vi "convert--chessboard_index to chess_square (chess notation).vi"(1 "chessboard_index":T4) -> (0 "chess_square (chess notation)":T1)   [LabVIEW 2020, in "core.lvlib"]
uses:
  core.lvlib
  core_data/chessboard_index.ctl
  core_data/chess_square--chess notation.ctl
  core_data/file--enum.ctl
  core_data/rank--enum.ctl
  core_data/core_data.lvlib
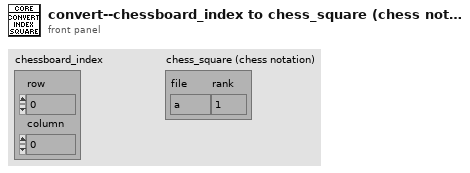
[diagram p1: front panel]
types:
  T1 = typedef "core.lvlib/core_data.lvlib/chess_square--chess notation.ctl" = cluster{"file":T2, "rank":T3}
  T2 = typedef "core.lvlib/core_data.lvlib/file--enum.ctl" = enum16{"a", "b", "c", "d", "e", "f", "g", "h"}
  T3 = typedef "core.lvlib/core_data.lvlib/rank--enum.ctl" = enum16{"1", "2", "3", "4", "5", "6", "7", "8"}
  T4 = typedef "core.lvlib/core_data.lvlib/chessboard_index.ctl" = cluster{"row":u8, "column":u8}
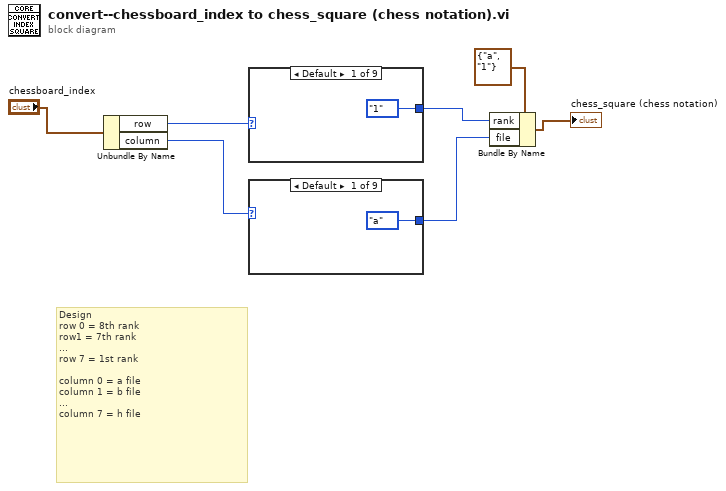
[diagram p0: block diagram]
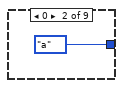
[diagram p2: hidden frame]
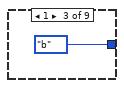
[diagram p3: hidden frame]
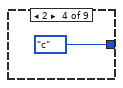
[diagram p4: hidden frame]
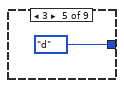
[diagram p5: hidden frame]
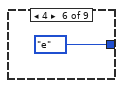
[diagram p6: hidden frame]
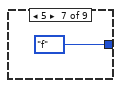
[diagram p7: hidden frame]
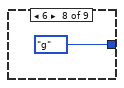
[diagram p8: hidden frame]
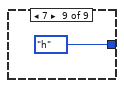
[diagram p9: hidden frame]
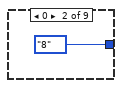
[diagram p10: hidden frame]
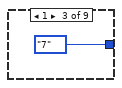
[diagram p11: hidden frame]
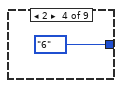
[diagram p12: hidden frame]
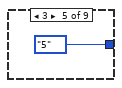
[diagram p13: hidden frame]
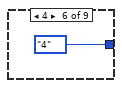
[diagram p14: hidden frame]
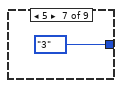
[diagram p15: hidden frame]
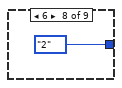
[diagram p16: hidden frame]
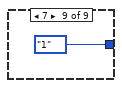
[diagram p17: hidden frame]
diagram:
  # "Design\nrow 0 = 8th rank\nrow1 = 7th rank\n...\nrow 7 = 1st rank\n\ncolumn 0 = a file\ncolumn 1 = b file\n...\ncolumn 7 = h file"
  n1 = Unbundle By Name("chessboard_index") -> ("row"=w4:u8, "column"=w2:u8)
  n2 = case shown="Default" w4 {
    tunnel: [rank--enum."1" ("rank") rank--enum."8" ("rank") rank--enum."7" ("rank") rank--enum."6" ("rank") rank--enum."5" ("rank") rank--enum."4" ("rank") rank--enum."3" ("rank") rank--enum."2" ("rank") rank--enum."1" ("rank")] -> w3
    frame Default {
    }
    frame 0 {
    }
    frame 1 {
    }
    frame 2 {
    }
    frame 3 {
    }
    frame 4 {
    }
    frame 5 {
    }
    frame 6 {
    }
    frame 7 {
    }
  }
  n3 = case shown="Default" w2 {
    tunnel: [file--enum."a" ("file") file--enum."a" ("file") file--enum."b" ("file") file--enum."c" ("file") file--enum."d" ("file") file--enum."e" ("file") file--enum."f" ("file") file--enum."g" ("file") file--enum."h" ("file")] -> w1
    frame Default {
    }
    frame 0 {
    }
    frame 1 {
    }
    frame 2 {
    }
    frame 3 {
    }
    frame 4 {
    }
    frame 5 {
    }
    frame 6 {
    }
    frame 7 {
    }
  }
  n4 = Bundle By Name(cluster=T1 {"file"=enum."a", "rank"=enum."1"} ("Chess square"), "rank"=w3, "file"=w1) -> (→"chess_square (chess notation)":T1)
